vi "Main.vi"() -> ()   [LabVIEW 2021]
doc: "This template is for the Queued Message Handler design pattern.\n\nThe Event Handling Loop generates messages based on user interface actions.\n\nThe Message Handling Loop processes messages generated by the Event Handling Loop, or by other messages. The messages are string values, so new messages can be added easily to the Message Cases case structure in the Message Handling Loop. Each message cluster can also provide an optional value for Message Data, which is a variant that can be converted to whatever message-specific data is required."
uses:
  TypeDef/MotorControlCluster.ctl
  controls/Status Lights.ctl
  controls/DAQ Refnums.ctl
  support/Message Queue/Enqueue Message (Single).vi
  <vilib>/Utility/error.llb/Error Cluster From Error Code.vi
  <vilib>/ErrorRing/Error Ring.xnode
  support/Message Queue/Message Queue.lvlib
  support/User Event - Stop/User Event - Stop.lvlib
panel:
  out "Motor Control Cluster":T1
  out "Pressure":dbl format="%0.2f"
  in  "Speed":dbl(knob) min=0.0 max=5.0 scale=0.0..5.0
  in  "Simulate":bool
  out "Status":string
  in  "Exit":bool
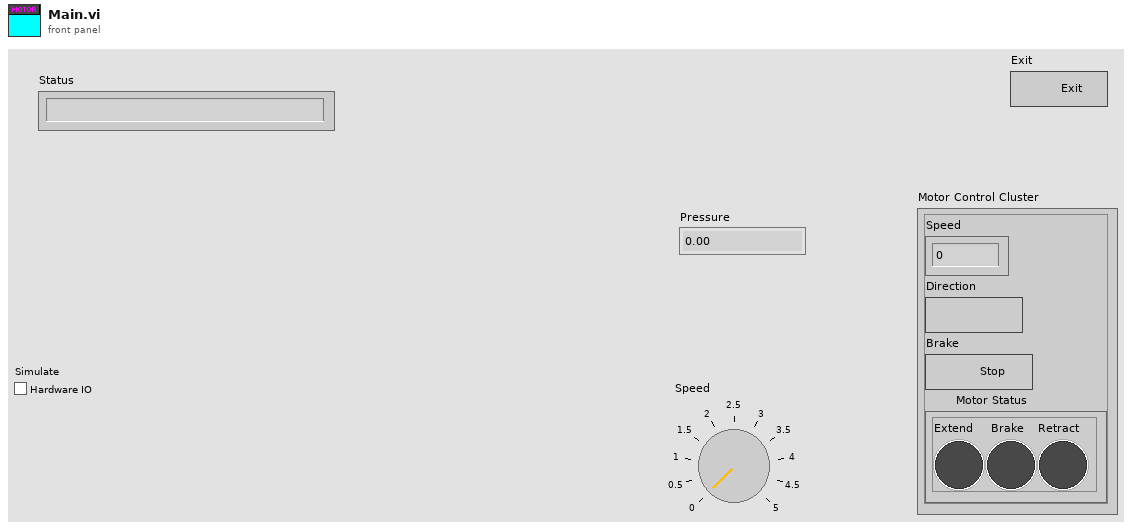
[diagram p1: front panel]
types:
  T1 = typedef "MotorControlCluster.ctl" = cluster{"Speed":dbl, "Direction":bool, "Brake":bool, "Motor Status":T2}
  T2 = typedef "Status Lights.ctl" = cluster{"Extend":bool, "Brake":bool, "Retract":bool}
  T3 = typedef "DAQ Refnums.ctl" = cluster{"Direction Ref":refnum<k21>, "Brake Ref":refnum<k21>, "Speed Ref":refnum<k21>, "Pressure Ref":refnum<k21>}
  T4 = typedef "Message Queue.lvlib/All Message Queues.ctl" = cluster{"UI":refnum<queue>}
  T5 = typedef "eventvkey.ctl" = enum16{"ASCII", "Enter", "Return", "Shift", "Ctrl", "Alt", "Cmd", "Opt", "Caps", "NumLock", "Clear", "Break", "Up", "Down", "Left", "Right", "Insert", "Delete", "Home", "End", "PageUp", "PageDown", "Escape", "Help", "Pause", "ScrollLock", "F1", "F2", "F3", "F4", "F5", "F6", "F7", "F8", "F9", "F10", "F11", "F12", "F13", "F14", "F15", "F16", "F17", "F18", "F19", "F20", "F21", "F22", "F23", "F24", "Play", "VolumeUp", "VolumeDown", "Mute", "Two Byte Char"}
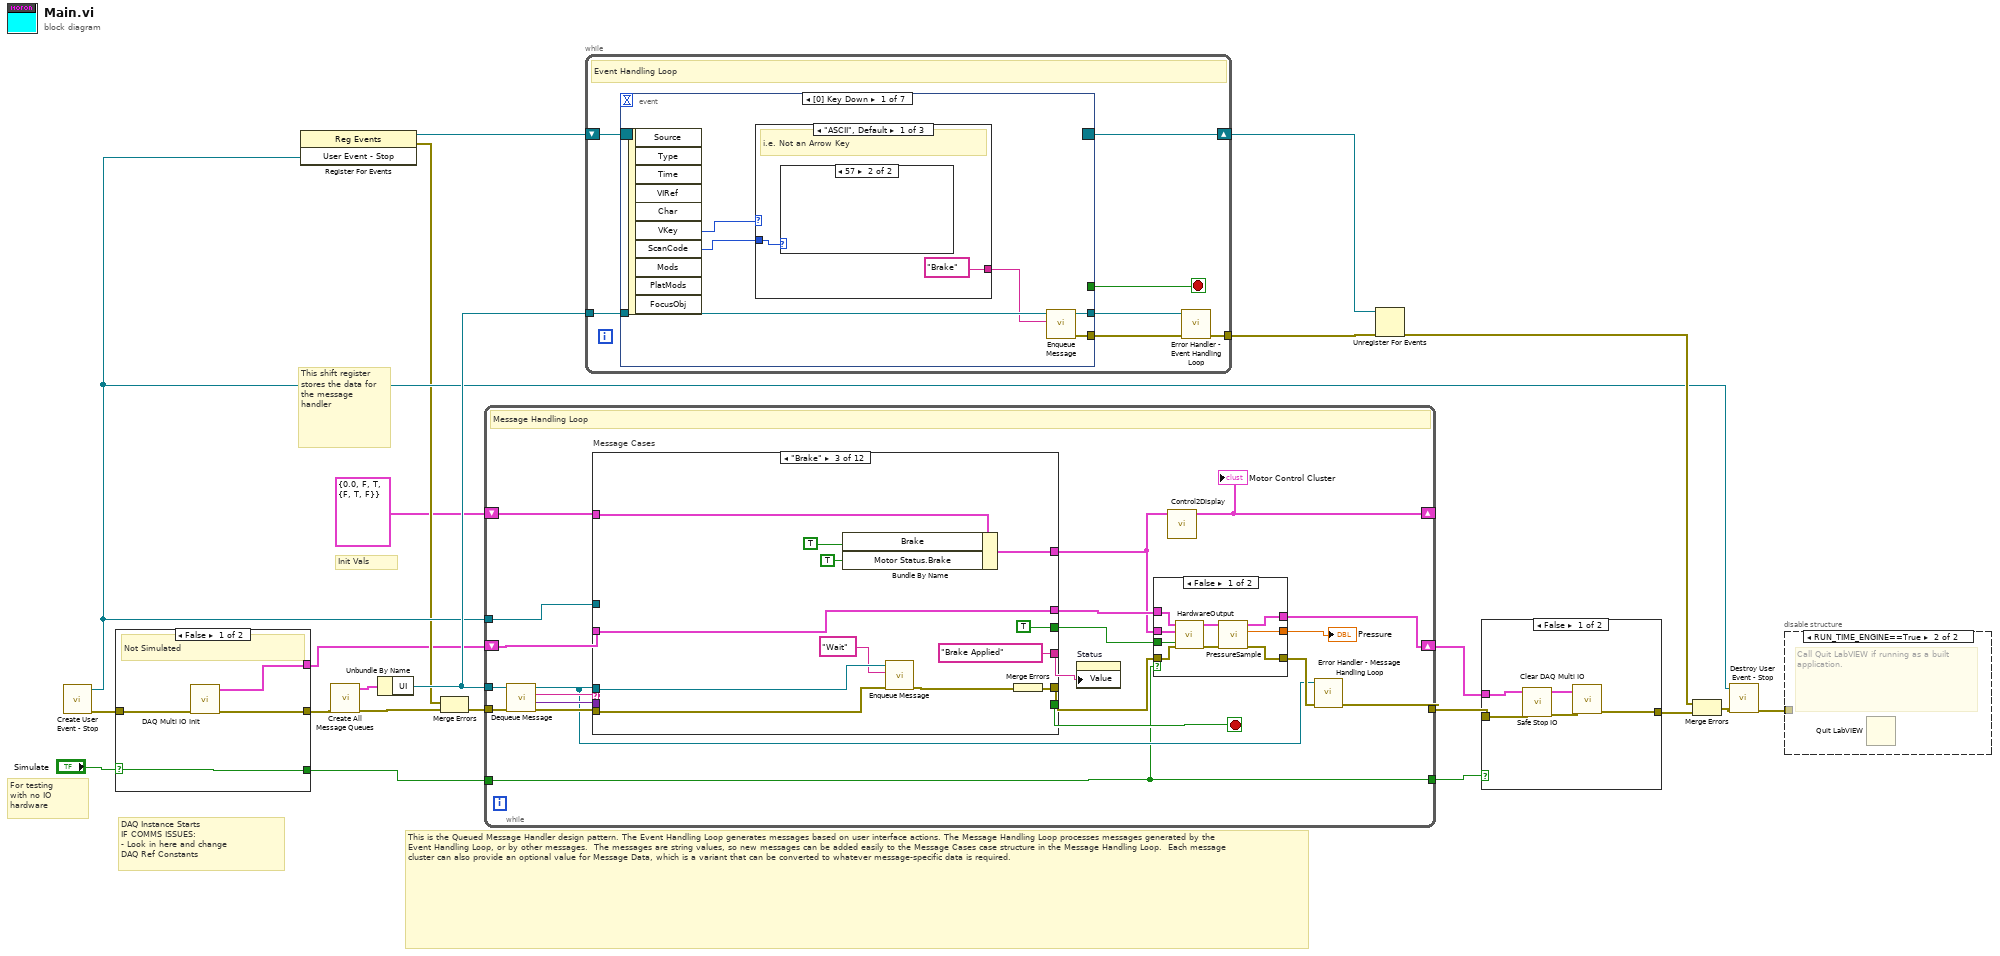
[diagram p0: block diagram]
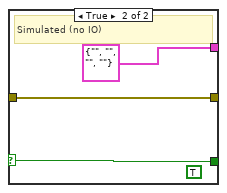
[diagram p3: hidden frame]
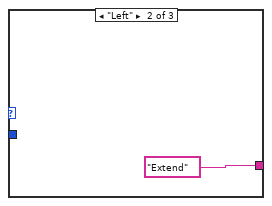
[diagram p6: hidden frame]
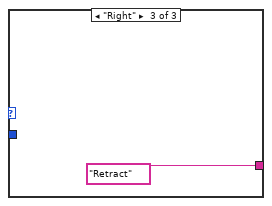
[diagram p7: hidden frame]
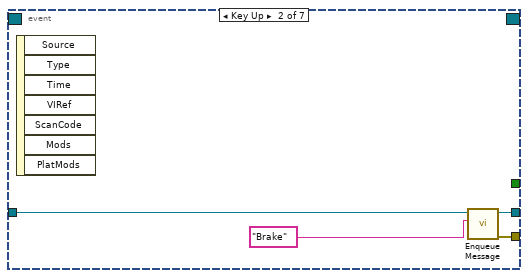
[diagram p8: hidden frame]
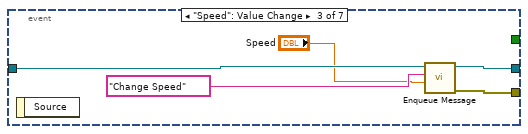
[diagram p9: hidden frame]
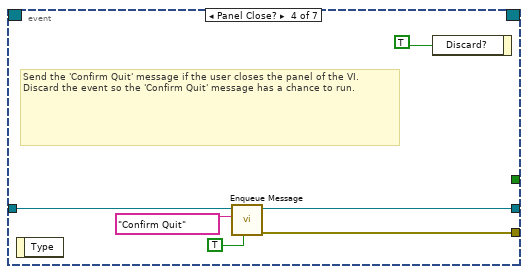
[diagram p10: hidden frame]
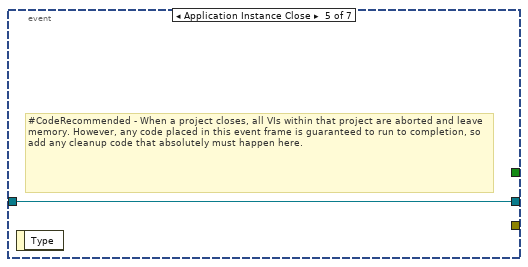
[diagram p11: hidden frame]
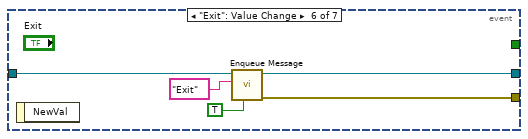
[diagram p12: hidden frame]
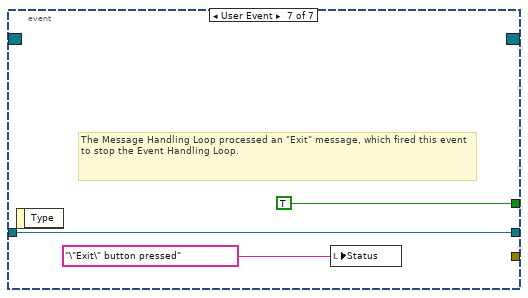
[diagram p13: hidden frame]
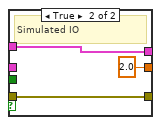
[diagram p14: hidden frame]
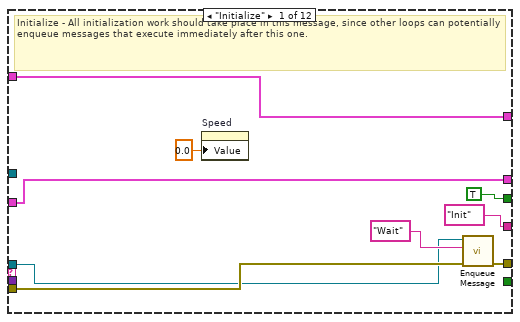
[diagram p15: hidden frame]
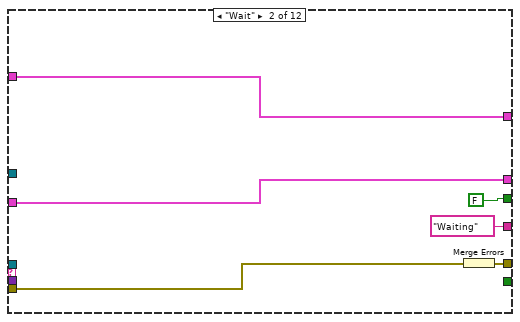
[diagram p16: hidden frame]
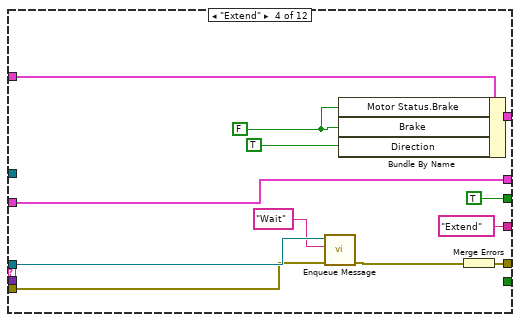
[diagram p17: hidden frame]
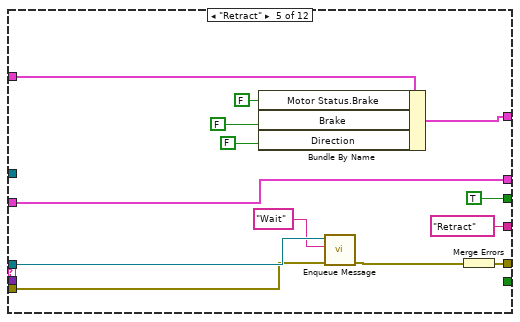
[diagram p18: hidden frame]
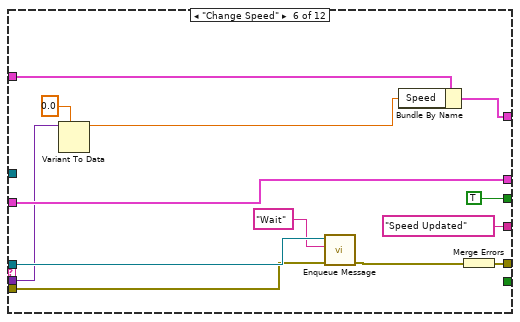
[diagram p19: hidden frame]
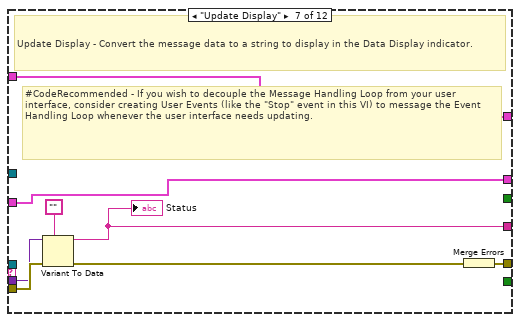
[diagram p20: hidden frame]
diagram:
  # "Init Vals"
  # "For testing \nwith no IO\nhardware"
  # "DAQ Instance Starts\nIF COMMS ISSUES:\n- Look in here and change\nDAQ Ref Constants"
  # "This is the Queued Message Handler design pattern. The Event Handling Loop generates messages based on user interface actions. The Message Handling Loop processes messages generated by the Event Handling Loop, or by other messages.  The messages are string values, so new messages can be added easily to the Message Cases case structure in the Message Handling Loop.  Each message cluster can also provide an optional value for Message Data, which is a variant that can be converted to whatever message-specific data is required."
  # "This shift register stores the data for the message handler"
  n1 = call "Create User Event - Stop.vi"() -> ("error out"=w10:errorcluster, "User Event - Stop"=w13:refnum<user-event>)  [unwired: 10 in]
  n2 = case shown="False" "Simulate" {
    selector: "Simulate" -> [w23 w27]
    tunnel: w10 -> [w26 w28]
    tunnel: [w25 w28] -> w9
    tunnel: [w24 T3 {"Direction Ref"="", "Brake Ref"="", "Speed Ref"="", "Pressure Ref"=""} ("DAQ Ref Cluster")] -> w8
    tunnel: [w23 w27] -> w2
    frame False {
      # "Not Simulated"
      n3 = call "DAQ Multi IO Init.vi"("error in"=w26) -> ("error out"=w25:errorcluster, "DAQ Ref Cluster"=w24:T3)  [unwired: 9 in]
    }
    frame True {
      (unwired) TRUE ("Visible")
      # "Simulated (no IO)"
    }
  }
  n4 = register-events(w13) -> (reference out=w14:refnum<event-registration>, error out=w11:errorcluster)  [unwired: 2 in]
  n5 = call "Create All Message Queues.vi"("error in (no error)"=w9) -> ("error out"=w22:errorcluster, "Message Queues out"=w21:T4)  [unwired: 9 in]
  n6 = Unbundle By Name(w21) -> ("UI"=w20:refnum<queue>)
  n7 = Merge Errors(w11, w22) -> (w12:errorcluster)
  n8 = while {
    tunnel: w20 -> [w44]
    shift-right: [w34] -> _
    shift-left: T1 {"Speed"=0.0, "Direction"=FALSE, "Brake"=TRUE, "Motor Status"={"Extend"=FALSE, "Brake"=TRUE, "Retract"=FALSE}} ("Motor Control Cluster") -> [w50]
    tunnel: w13 -> [w48]
    tunnel: w12 -> [w38]
    tunnel: [w43] -> w5
    shift-right: [w33] -> w4
    shift-left: w8 -> [w37]
    tunnel: [w31] -> w1
    tunnel: w2 -> [w31]
    stop <- w49 stop-if-true
    # "Message Handling Loop"
    n9 = call "Dequeue Message.vi"("error in (no error)"=w38, "Message Queue"=w44) -> ("error out"=w47:errorcluster, "Message Data"=w45:variant, "Message"=w46:string, "dup Message Queue"=w32:refnum<queue>)  [unwired: 6 in]
    n10 = case "Message Cases" shown="\"Brake\"" w46 {
      selector: w46 -> [_ _ _ _ _ _ _ _ _ _ _ w174]
      tunnel: w32 -> [w68 _ w82 w95 w107 w121 _ _ w149 _ w171 _]
      tunnel: w47 -> [w70 w74 w81 w94 w106 w120 w133 w144 w153 w158 w164 _]
      tunnel: [w71 w76 w89 w101 w114 w127 w134 w138 w151 w156 w167 w175] -> w40
      tunnel: w50 -> [w65 w77 w84 w96 w109 w122 w135 w143 w152 w157 w170 w176]
      tunnel: [w65 w77 w85 w97 w110 w123 w135 w143 w152 w157 w170 w176] -> w30
      tunnel: [_ _ _ _ _ _ _ _ _ _ TRUE _] -> w49
      tunnel: w45 -> [_ _ _ _ _ w117 w132 w142 _ _ w161 _]
      tunnel: w48 -> [_ _ _ _ _ _ _ _ _ _ w166 _]
      tunnel: w37 -> [w64 w75 w88 w100 w113 w126 w129 w136 w145 w154 w159 w172]
      tunnel: ["Init" ("Initial Message") "Waiting" ("Initial Message") "Brake Applied" ("Initial Message") "Extend" ("Initial Message") "Retract" ("Initial Message") "Speed Updated" ("Initial Message") w128 "ERROR" ("Initial Message") "Quitting" ("Initial Message") "Copy" ("Initial Message") "Exit" ("Initial Message") "ERROR: INVALID MESSAGE" ("Initial Message")] -> w42
      tunnel: [w64 w75 w88 w100 w113 w126 w129 w136 w145 w154 w159 w172] -> w41
      tunnel: [TRUE FALSE TRUE TRUE TRUE TRUE _ _ _ _ _ _] -> w39
      frame "Initialize" {
        # "Initialize - All initialization work should take place in this message, since other loops can potentially enqueue messages that execute immediately after this one."
        n11 = property on="Speed" class="Knob (strict)"("Value"=0.0 ("Speed")) -> ()  [unwired: 2 in, 2 out]
        n12 = call-poly "Enqueue Message.vi"("error in (no error)"=w70, "Message"="Wait", "Message Queue"=w68) -> ("error out"=w71:errorcluster)  [unwired: 7 in, 1 out]
      }
      frame "Wait" {
        n13 = Merge Errors(w74) -> (w76:errorcluster)
      }
      frame "Brake" {
        n14 = Bundle By Name(cluster=w84, "Brake"=TRUE, "Motor Status.Brake"=TRUE) -> (w85:T1)
        n15 = call-poly "Enqueue Message.vi"("error in (no error)"=w81, "Message"="Wait", "Message Queue"=w82) -> ("error out"=w80:errorcluster)  [unwired: 7 in, 1 out]
        n16 = Merge Errors(w80) -> (w89:errorcluster)
      }
      frame "Extend" {
        w90 = FALSE ("Brake")
        n17 = call-poly "Enqueue Message.vi"("error in (no error)"=w94, "Message"="Wait", "Message Queue"=w95) -> ("error out"=w93:errorcluster)  [unwired: 7 in, 1 out]
        n18 = Bundle By Name(cluster=w96, "Motor Status.Brake"=w90, "Brake"=w90, "Direction"=TRUE) -> (w97:T1)
        n19 = Merge Errors(w93) -> (w101:errorcluster)
      }
      frame "Retract" {
        n20 = Bundle By Name(cluster=w109, "Motor Status.Brake"=FALSE, "Brake"=FALSE, "Direction"=FALSE) -> (w110:T1)
        n21 = call-poly "Enqueue Message.vi"("error in (no error)"=w106, "Message"="Wait", "Message Queue"=w107) -> ("error out"=w105:errorcluster)  [unwired: 7 in, 1 out]
        n22 = Merge Errors(w105) -> (w114:errorcluster)
      }
      frame "Change Speed" {
        n23 = Variant To Data(type=0.0 ("Speed"), Variant=w117) -> (data=w115:dbl)  [unwired: 1 in, 1 out]
        n24 = call-poly "Enqueue Message.vi"("error in (no error)"=w120, "Message"="Wait", "Message Queue"=w121) -> ("error out"=w119:errorcluster)  [unwired: 7 in, 1 out]
        n25 = Bundle By Name(cluster=w122, "Speed"=w115) -> (w123:T1)
        n26 = Merge Errors(w119) -> (w127:errorcluster)
      }
      frame "Update Display" {
        # "#CodeRecommended - If you wish to decouple the Message Handling Loop from your user interface, consider creating User Events (like the \"Stop\" event in this VI) to message the Event Handling Loop whenever the user interface needs updating."
        # "Update Display - Convert the message data to a string to display in the Data Display indicator."
        n27 = Variant To Data(error in=w133, type="", Variant=w132) -> (data=w128:string, error out=w130:errorcluster)
        "Status" <- w128
        n28 = Merge Errors(w130) -> (w134:errorcluster)
      }
      frame "Error" {
        # "#CodeRecommended - If you ever change the name of this \"Error\" message, you'll need to update the name in the Check Loop Error.vi as well."
        # "#CodeRecommended - Consider creating a system for logging errors in some way. These errors are for notification purposes only. Handling of specific errors should be performed in the message frames that generated the error."
        # "Error - Display an error dialog. This message is sent by the \"Error Handler\" VIs at the end of other loops in this application."
        n29 = Variant To Data(error in=w144, type=errorcluster {"status"=FALSE, "code"=0, "source"=""} ("error constant"), Variant=w142) -> (data=w140:errorcluster, error out=w139:errorcluster)
        n30 = call <vilib>:"Simple Error Handler.vi"("error in (no error)"=w140) -> ()  [unwired: 4 in, 5 out]
        n31 = Merge Errors(w139) -> (w138:errorcluster)
      }
      frame "Confirm Quit" {
        # "#CodeNeeded - If you want to provide an \"Are you sure\" dialog (or some other notification) before the application exits, place that code here. This message is typically sent from a Panel Close? event."
        # "Confirm Quit - Message that can confirm whether or not the user wants to exit the application."
        n32 = call-poly "Enqueue Message.vi"("Priority Message? (F)"=TRUE, "error in (no error)"=w153, "Message"="Exit", "Message Queue"=w149) -> ("error out"=w150:errorcluster)  [unwired: 6 in, 1 out]
        n33 = Merge Errors(w150) -> (w151:errorcluster)
      }
      frame "---Copy This Frame---" {
        # "Duplicate this frame when creating new messages.  Change this comment in the duplicated frame to describe this message."
        n34 = Merge Errors(w158) -> (w156:errorcluster)
      }
      frame "Exit" {
        # "Stop the VI"
        # "Release the message queue reference"
        # "#CodeNeeded - Add any required cleanup code here. Note that if 'Exit' was called as a result of an error, an error dialog will be displayed. Add any custom error handling for an 'Exit' condition here as well."
        # "Exit - Exit the application."
        n35 = Variant To Data(type=errorcluster {"status"=FALSE, "code"=0, "source"=""} ("error constant"), Variant=w161) -> (data=w162:errorcluster)  [unwired: 1 in, 1 out]
        n36 = call <vilib>:"Simple Error Handler.vi"("error in (no error)"=w162) -> ()  [unwired: 4 in, 5 out]
        n37 = call "Fire User Event - Stop.vi"("User Event - Stop"=w166) -> ("error out"=w165:errorcluster)  [unwired: 10 in]
        n38 = Release Queue(queue=w171, error in (no error)=w164) -> (error out=w168:errorcluster)  [unwired: 1 in, 2 out]
        n39 = Merge Errors(w165, w168) -> (w167:errorcluster)
      }
      frame Default {
        # "'Default' case only runs if there is a message that isn't defined in any of the other cases.  Output a programming error."
        n40 = xnode "Error Ring"("parameter 0"=w174) -> ("error out"=w175:errorcluster)
      }
    }
    n41 = property on="Status" class="Str"("Value"=w42) -> ()  [unwired: 2 in, 2 out]
    n42 = case shown="False" w31 {
      tunnel: w41 -> [w59 w62]
      tunnel: w40 -> [w58 w61]
      tunnel: w39 -> [w57 _]
      tunnel: w30 -> [w56 _]
      tunnel: [w53 w61] -> w36
      tunnel: [w52 2.0 ("Detected Voltage")] -> w35
      tunnel: [w51 w62] -> w33
      frame False {
        n43 = call "HardwareOutput.vi"("error in"=w58, "Update Outputs"=w57, "Motor Control Cluster"=w56, "DAQREFs in"=w59) -> ("error out"=w55:errorcluster, "DAQREFs out"=w54:T3)  [unwired: 6 in]
        n44 = call "PressureSample.vi"("error in (no error)"=w55, "DAQREFS"=w54) -> ("error out"=w53:errorcluster, "Detected Voltage"=w52:dbl, "DAQREFs"=w51:T3)  [unwired: 7 in]
      }
      frame True {
        # "Simulated IO"
      }
    }
    "Pressure" <- w35
    n45 = call "Control2Display.vi"("Motor Control Cluster"=w30) -> ("Motor Control Cluster"=w34:T1)  [unwired: 10 in]
    "Motor Control Cluster" <- w34
    n46 = call "Error Handler - Message Handling Loop.vi"("error in (no error)"=w36, "Message Queue"=w32) -> ("dup error in"=w43:errorcluster)  [unwired: 8 in, 1 out]
  }
  n47 = while {
    tunnel: w20 -> [w190]
    shift-right: [w188] -> w17
    shift-left: w14 -> [w189]
    tunnel: [w184] -> w15
    stop <- w186 stop-if-true
    # "Event Handling Loop"
    n48 = event shown="[0] Key Down" {
      selector: w189 -> [_ _ _ _ _ _ _]
      dyn-events: [_ _ _ _ _ _ _] -> w188
      timeout: _ -> [_ _ _ _ _ _ _]
      tunnel: [_ _ _ _ _ _ TRUE ("Discard?")] -> w186
      tunnel: w190 -> [w196 w204 w209 w215 w216 w221 w224]
      tunnel: [w194 w202 w206 w214 _ w220 _] -> w187
      tunnel: [w195 w203 w208 w213 w216 w219 w224] -> w185
      event Key Down {
        n49 = event-data() -> ("VKey"=w193:T5, "ScanCode"=w192:i16)  [unwired: 1 in, 8 out]
        n50 = case shown="\"ASCII\", Default" w193 {
          tunnel: w192 -> [w198 _ _]
          tunnel: ["Brake" ("Message") "Extend" ("Message") "Retract" ("Message")] -> w191
          frame "ASCII", Default {
            # "i.e. Not an Arrow Key"
            n51 = case shown="57" w198 {
              frame Default {
              }
              frame 57 {
              }
            }
          }
          frame "Left" {
          }
          frame "Right" {
          }
        }
        n52 = call-poly "Enqueue Message.vi"("Message"=w191, "Message Queue"=w196) -> ("error out"=w194:errorcluster, "dup Message Queue"=w195:refnum<queue>)  [unwired: 8 in]
      }
      event Key Up {
        n53 = event-data() -> ()  [unwired: 1 in, 7 out]
        n54 = call-poly "Enqueue Message.vi"("Message"="Brake", "Message Queue"=w204) -> ("error out"=w202:errorcluster, "dup Message Queue"=w203:refnum<queue>)  [unwired: 8 in]
      }
      event "Speed": Value Change {
        n55 = event-data() -> ()  [unwired: 1 in, 1 out]
        n56 = call-poly "Enqueue Message.vi"("Message Data"="Speed", "Message"="Change Speed", "Message Queue"=w209) -> ("error out"=w206:errorcluster, "dup Message Queue"=w208:refnum<queue>)  [unwired: 7 in]
      }
      event Panel Close? {
        # "Send the 'Confirm Quit' message if the user closes the panel of the VI. Discard the event so the 'Confirm Quit' message has a chance to run."
        n57 = event-data() -> ()  [unwired: 1 in, 1 out]
        n58 = call-poly "Enqueue Message.vi"("Priority Message? (F)"=TRUE, "Message"="Confirm Quit", "Message Queue"=w215) -> ("error out"=w214:errorcluster, "dup Message Queue"=w213:refnum<queue>)  [unwired: 7 in]
        n59 = event-data("Discard?"=TRUE) -> ()  [unwired: 1 in, 1 out]
      }
      event Application Instance Close {
        # "#CodeRecommended - When a project closes, all VIs within that project are aborted and leave memory. However, any code placed in this event frame is guaranteed to run to completion, so add any cleanup code that absolutely must happen here."
        n60 = event-data() -> ()  [unwired: 1 in, 1 out]
      }
      event "Exit": Value Change {
        n61 = event-data() -> ()  [unwired: 1 in, 1 out]
        n62 = call-poly "Enqueue Message.vi"("Priority Message? (F)"=TRUE, "Message"="Exit", "Message Queue"=w221) -> ("error out"=w220:errorcluster, "dup Message Queue"=w219:refnum<queue>)  [unwired: 7 in]
      }
      event User Event {
        # "The Message Handling Loop processed an \"Exit\" message, which fired this event to stop the Event Handling Loop."
        n63 = event-data() -> ()  [unwired: 1 in, 1 out]
        n64 = local write "Status"("\"Exit\" button pressed" ("VI Stopped")) -> ()
      }
    }
    n65 = call "Error Handler - Event Handling Loop.vi"("error in (no error)"=w187, "Message Queue"=w185) -> ("dup error in"=w184:errorcluster)  [unwired: 8 in, 1 out]
  }
  n66 = Unregister For Events(event registration refnum=w17, error in=w15) -> (error out=w18:errorcluster)
  n67 = case shown="False" w1 {
    tunnel: [w229 w230] -> w3
    tunnel: w4 -> [w228 _]
    tunnel: w5 -> [w227 w230]
    frame False {
      n68 = call "Safe Stop IO.vi"("error in"=w227, "DAQ Ref Cluster"=w228) -> ("error out"=w225:errorcluster, "DAQ Ref Cluster Out"=w226:T3)  [unwired: 8 in]
      n69 = call "Clear DAQ Multi IO.vi"("error in"=w225, "DAQ Ref"=w226) -> ("error out"=w229:errorcluster)  [unwired: 9 in]
    }
    frame True {
    }
  }
  n70 = Merge Errors(w18, w3) -> (w19:errorcluster)
  n71 = call "Destroy User Event - Stop.vi"("error in (no error)"=w19, "User Event - Stop"=w13) -> ("error out"=w16:errorcluster)  [unwired: 9 in]
  n72 = disable-structure shown="RUN_TIME_ENGINE==True" {
    disable-tunnel: w16 -> [_ _]
    frame condition #0 (active) {
    }
    frame condition #1 {
      # "Call Quit LabVIEW if running as a built application."
      n73 = Quit LabVIEW() -> ()  [unwired: 1 in]
    }
  }
